vi "CoffeMachineMain.vi"() -> ()   [LabVIEW 2021]
panel:
  in  "Coffe":dbl(slide) scale=0.0..100.0
  in  "Tea":dbl(slide) scale=0.0..100.0
  in  "Water":dbl(slide) scale=0.0..100.0
  in  "İçicek":i64(knob) scale=0.0..2.0
  in  "Sürahi":bool
  in  "Kupa":bool
  out "Preparation":bool
  out "Grinding":bool
  out "Brewing":bool
  out "Distillation":bool
  out "Heating":bool
  out "Cleaning":bool
  out "Status":string
  in  "Power off":bool
  # "Control"
  # "Indıcator"
  # "Tea"
  # "Water"
  # "Coffe"
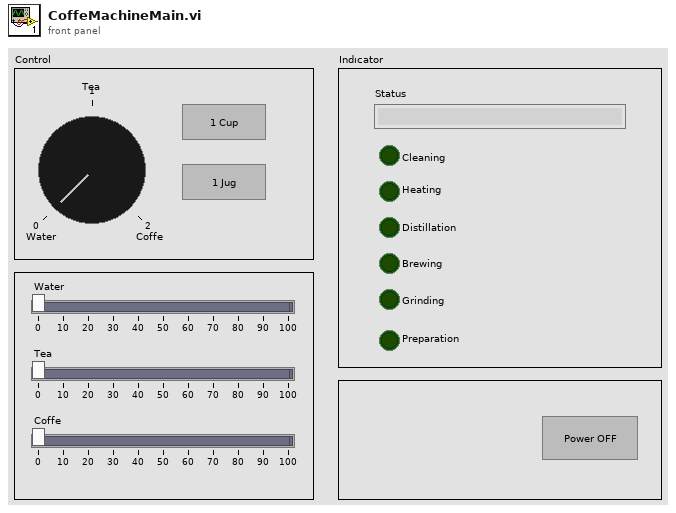
[diagram p1: front panel]
types:
  T1 = cluster{"element":string, "Message Data":variant}
  T2 = cluster{"Çay":dbl, "Su":dbl, "Kahve":dbl, "Power Status":bool}
  T3 = enum8{"Enabled", "Disabled", "Disabled and Grayed Out"}
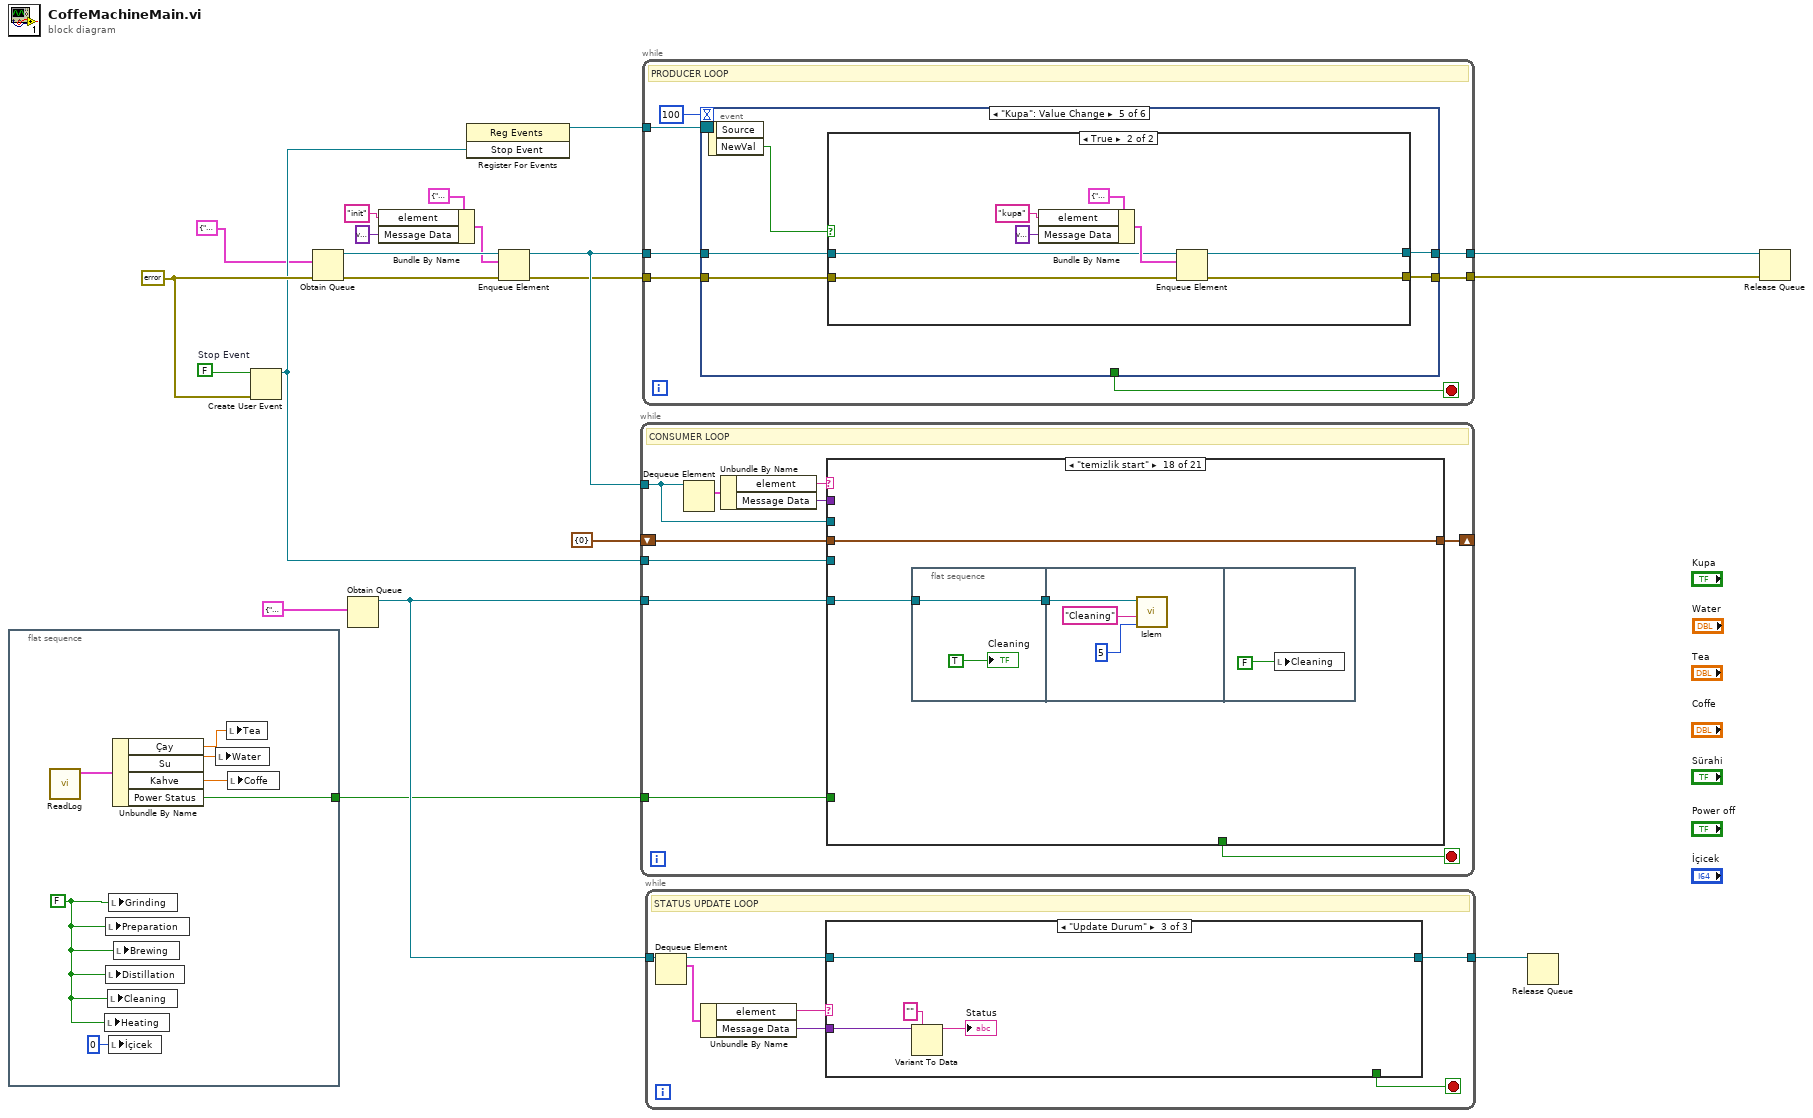
[diagram p0: block diagram]
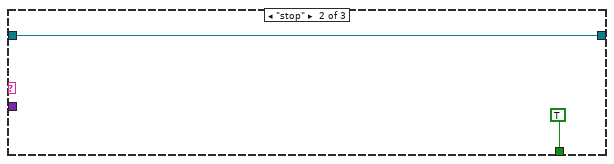
[diagram p3: hidden frame]
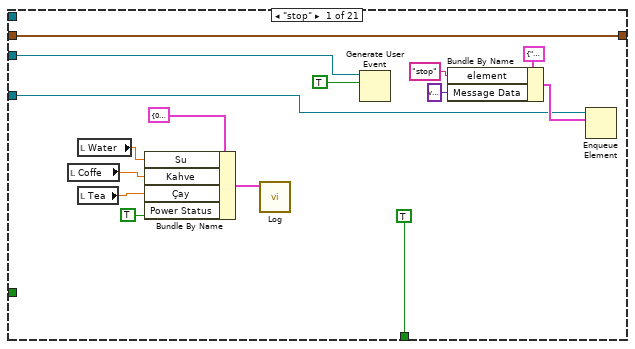
[diagram p4: hidden frame]
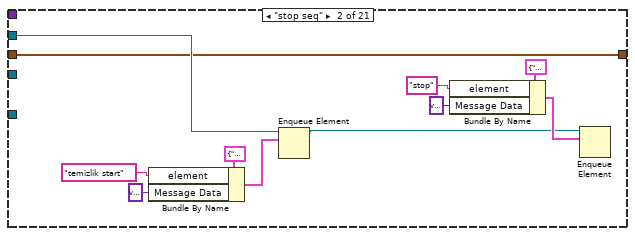
[diagram p5: hidden frame]
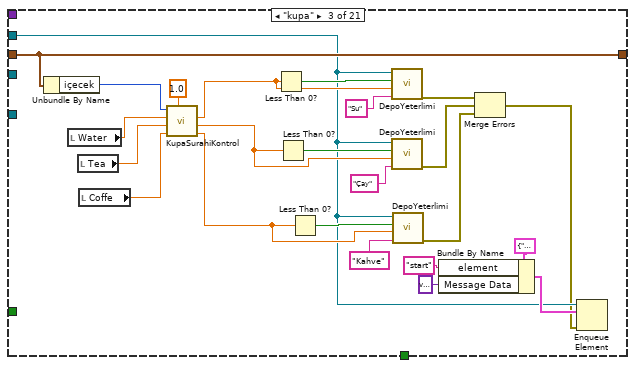
[diagram p6: hidden frame]
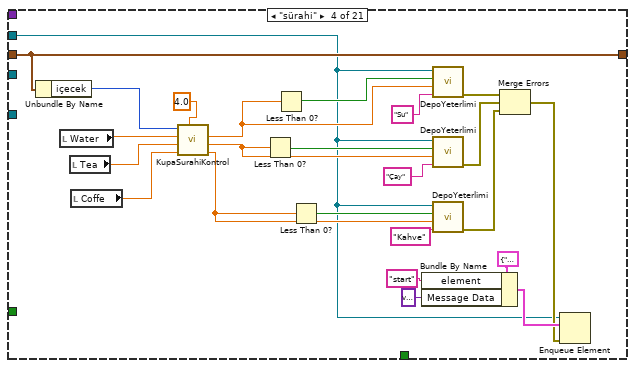
[diagram p7: hidden frame]
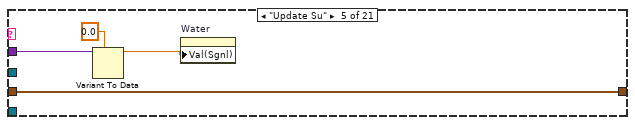
[diagram p8: hidden frame]
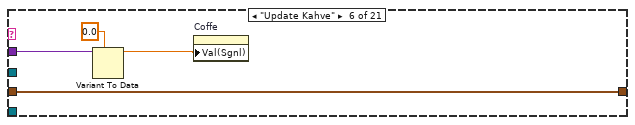
[diagram p9: hidden frame]
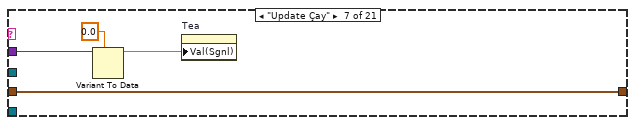
[diagram p10: hidden frame]
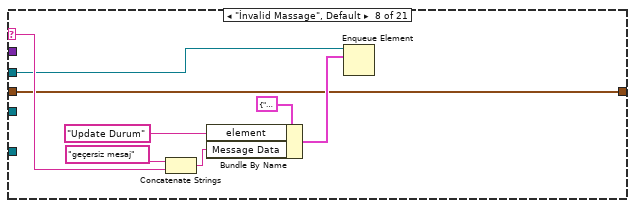
[diagram p11: hidden frame]
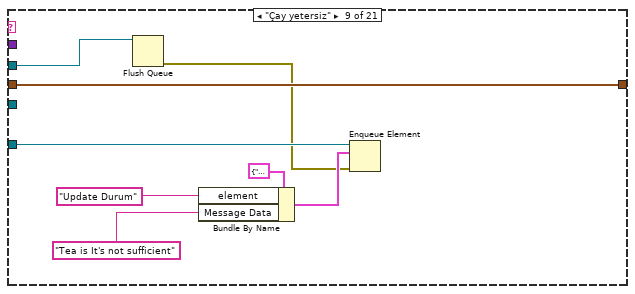
[diagram p12: hidden frame]
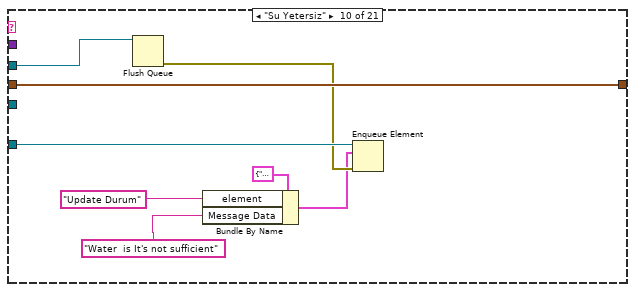
[diagram p13: hidden frame]
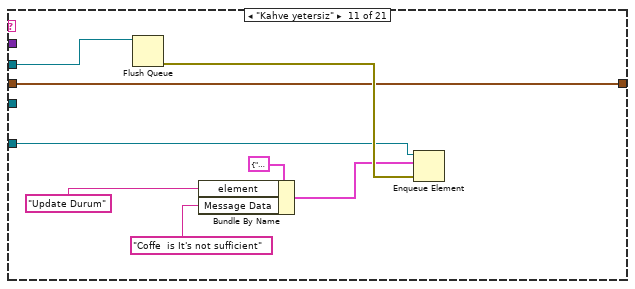
[diagram p14: hidden frame]
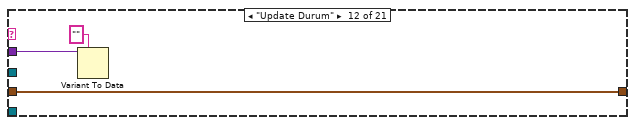
[diagram p15: hidden frame]
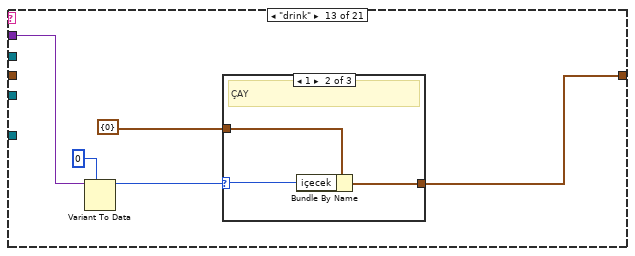
[diagram p16: hidden frame]
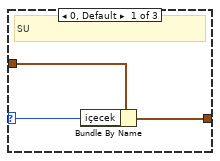
[diagram p17: hidden frame]
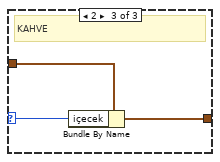
[diagram p18: hidden frame]
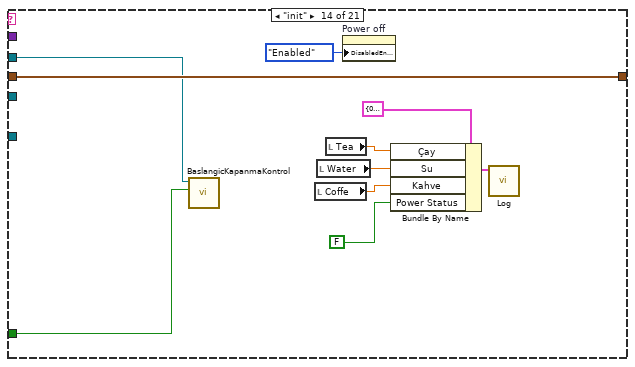
[diagram p19: hidden frame]
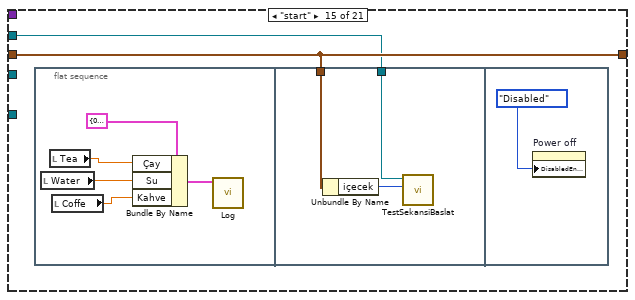
[diagram p20: hidden frame]
diagram:
  w13 = FALSE  # Stop Event
  w14 = errorcluster {"status"=FALSE, "code"=0, "source"=""} ("error in (no error)")
  n1 = flat-sequence {
    tunnel: [w23] -> w1
    frame #0 {
      w22 = FALSE ("Öğütme")
      n2 = call "ReadLog.vi"() -> ("data out"=w27:T2)  [unwired: 11 in]
      n3 = local write "Heating"(w22) -> ()
      n4 = local write "Preparation"(w22) -> ()
      n5 = local write "Distillation"(w22) -> ()
      n6 = local write "Cleaning"(w22) -> ()
      n7 = local write "Grinding"(w22) -> ()
      n8 = local write "İçicek"(i64 0 ("İçicek")) -> ()
      n9 = Unbundle By Name(w27) -> ("Çay"=w25:dbl, "Su"=w26:dbl, "Kahve"=w24:dbl, "Power Status"=w23:bool)
      n10 = local write "Brewing"(w22) -> ()
      n11 = local write "Water"(w26) -> ()
      n12 = local write "Tea"(w25) -> ()
      n13 = local write "Coffe"(w24) -> ()
    }
  }
  n14 = Create User Event(user event datatype=w13, error in=w14) -> (user event=w11:refnum<user-event>)  [unwired: 1 out]
  n15 = Obtain Queue(element data type=T1 {"element"="", "Message Data"=variant}, error in (no error)=w14) -> (queue out=w18:refnum<queue>, error out=w17:errorcluster)  [unwired: 3 in, 1 out]
  n16 = Obtain Queue(element data type=T1 {"element"="", "Message Data"=variant}) -> (queue out=w4:refnum<queue>)  [unwired: 4 in, 2 out]
  n17 = Bundle By Name(cluster=T1 {"element"="", "Message Data"=variant}, "element"="init", "Message Data"=variant) -> (w8:T1)
  n18 = register-events(w11) -> (reference out=w12:refnum<event-registration>)  [unwired: 2 in, 1 out]
  n19 = Enqueue Element(queue=w18, element=w8, error in (no error)=w17) -> (queue out=w16:refnum<queue>, error out=w15:errorcluster)  [unwired: 1 in, 1 out]
  n20 = while {
    tunnel: w16 -> [w30]
    tunnel: w11 -> [w37]
    shift-right: [w32] -> _
    shift-left: cluster{"içecek":i64} {"içecek"=0} -> [w33]
    tunnel: w4 -> [w29]
    tunnel: w1 -> [w28]
    stop <- w36 stop-if-true
    # "CONSUMER LOOP"
    n21 = Dequeue Element(queue=w30) -> (element=w35:T1)  [unwired: 2 in, 3 out]
    n22 = Unbundle By Name(w35) -> ("element"=w34:string, "Message Data"=w31:variant)
    n23 = case shown="\"temizlik start\"" w34 {
      selector: w34 -> [_ _ _ _ _ _ _ w128 _ _ _ _ _ _ _ _ _ _ _ _ _]
      tunnel: w37 -> [w51 _ _ _ _ _ _ _ _ _ _ _ _ _ _ _ _ _ _ _ _]
      tunnel: [TRUE _ _ _ _ _ _ _ _ _ _ _ _ _ _ _ _ _ _ _ _] -> w36
      tunnel: w33 -> [w49 w53 w87 w111 w113 w117 w121 w124 w136 w143 w149 w156 _ w182 w184 w196 w203 w212 w223 w233 w242]
      tunnel: [w49 w53 w87 w111 w113 w117 w121 w124 w136 w143 w149 w156 w160 w182 w184 w196 w203 w212 w223 w233 w242] -> w32
      tunnel: w31 -> [_ _ _ _ w115 w119 w123 _ _ _ _ w158 w163 _ _ _ _ _ _ _ _]
      tunnel: w30 -> [_ w54 w65 w88 _ _ _ w126 w139 w147 w155 _ _ w179 w183 _ _ _ _ _ _]
      tunnel: w29 -> [w44 _ _ _ _ _ _ _ w134 w142 w148 _ _ _ _ w194 w204 w213 w221 w231 w241]
      tunnel: w28 -> [_ _ _ _ _ _ _ _ _ _ _ _ _ w180 _ _ _ _ _ _ _]
      frame "stop" {
        n24 = local read "Coffe"() -> (w40:dbl)
        n25 = local read "Water"() -> (w42:dbl)
        n26 = local read "Tea"() -> (w41:dbl)
        n27 = Bundle By Name(cluster=T2 {"Çay"=0.0, "Su"=0.0, "Kahve"=0.0, "Power Status"=FALSE}, "Su"=w42, "Kahve"=w40, "Çay"=w41, "Power Status"=TRUE) -> (w38:T2)
        n28 = call "Log.vi"("Data"=w38) -> ()  [unwired: 11 in]
        n29 = Generate User Event(user event=w51, event data cluster=TRUE ("event data")) -> ()  [unwired: 2 in, 2 out]
        n30 = Bundle By Name(cluster=T1 {"element"="", "Message Data"=variant}, "element"="stop", "Message Data"=variant) -> (w47:T1)
        n31 = Enqueue Element(queue=w44, element=w47) -> ()  [unwired: 2 in, 3 out]
      }
      frame "stop seq" {
        n32 = Bundle By Name(cluster=T1 {"element"="", "Message Data"=variant}, "element"="temizlik start", "Message Data"=variant) -> (w63:T1)
        n33 = Enqueue Element(queue=w54, element=w63) -> (queue out=w55:refnum<queue>)  [unwired: 2 in, 2 out]
        n34 = Bundle By Name(cluster=T1 {"element"="", "Message Data"=variant}, "element"="stop", "Message Data"=variant) -> (w56:T1)
        n35 = Enqueue Element(queue=w55, element=w56) -> ()  [unwired: 2 in, 3 out]
      }
      frame "kupa" {
        n36 = Unbundle By Name(w87) -> ("içecek"=w85:i64)
        n37 = local read "Water"() -> (w86:dbl)
        n38 = local read "Tea"() -> (w84:dbl)
        n39 = local read "Coffe"() -> (w83:dbl)
        n40 = call "KupaSurahiKontrol.vi"("Çarpan"=1.0, "Kahve"=w83, "Çay"=w84, "Su"=w86, "içicek"=w85) -> ("Kahve çıkış"=w73:dbl, "Çay çıkış"=w76:dbl, "Su çıkış"=w80:dbl)  [unwired: 4 in]
        n41 = Less Than 0?(x=w80) -> (x < 0?=w81:bool)
        n42 = Less Than 0?(x=w76) -> (x < 0?=w77:bool)
        n43 = Less Than 0?(x=w73) -> (x < 0?=w74:bool)
        n44 = call "DepoYeterlimi.vi"("Element"="Su", "Massage Data"=w80, "Yeterlimi?"=w81, "queue out"=w65) -> ("error out"=w72:errorcluster)  [unwired: 7 in]
        n45 = call "DepoYeterlimi.vi"("Element"="Çay", "Massage Data"=w76, "Yeterlimi?"=w77, "queue out"=w65) -> ("error out"=w71:errorcluster)  [unwired: 7 in]
        n46 = call "DepoYeterlimi.vi"("Element"="Kahve", "Massage Data"=w73, "Yeterlimi?"=w74, "queue out"=w65) -> ("error out"=w70:errorcluster)  [unwired: 7 in]
        n47 = Bundle By Name(cluster=T1 {"element"="", "Message Data"=variant}, "element"="start", "Message Data"=variant) -> (w69:T1)
        n48 = Merge Errors(w72, w71, w70) -> (w64:errorcluster)
        n49 = Enqueue Element(queue=w65, element=w69, error in (no error)=w64) -> ()  [unwired: 1 in, 3 out]
      }
      frame "sürahi" {
        n50 = Unbundle By Name(w111) -> ("içecek"=w110:i64)
        n51 = local read "Water"() -> (w108:dbl)
        n52 = local read "Tea"() -> (w107:dbl)
        n53 = local read "Coffe"() -> (w106:dbl)
        n54 = call "KupaSurahiKontrol.vi"("Çarpan"=4.0 ("x"), "Kahve"=w106, "Çay"=w107, "Su"=w108, "içicek"=w110) -> ("Kahve çıkış"=w97:dbl, "Çay çıkış"=w100:dbl, "Su çıkış"=w104:dbl)  [unwired: 4 in]
        n55 = Less Than 0?(x=w100) -> (x < 0?=w101:bool)
        n56 = Less Than 0?(x=w104) -> (x < 0?=w105:bool)
        n57 = Less Than 0?(x=w97) -> (x < 0?=w98:bool)
        n58 = Bundle By Name(cluster=T1 {"element"="", "Message Data"=variant}, "element"="start", "Message Data"=variant) -> (w93:T1)
        n59 = call "DepoYeterlimi.vi"("Element"="Su" ("element"), "Massage Data"=w104, "Yeterlimi?"=w105, "queue out"=w88) -> ("error out"=w96:errorcluster)  [unwired: 7 in]
        n60 = call "DepoYeterlimi.vi"("Element"="Çay" ("element"), "Massage Data"=w100, "Yeterlimi?"=w101, "queue out"=w88) -> ("error out"=w95:errorcluster)  [unwired: 7 in]
        n61 = call "DepoYeterlimi.vi"("Element"="Kahve", "Massage Data"=w97, "Yeterlimi?"=w98, "queue out"=w88) -> ("error out"=w94:errorcluster)  [unwired: 7 in]
        n62 = Merge Errors(w96, w95, w94) -> (w89:errorcluster)
        n63 = Enqueue Element(queue=w88, element=w93, error in (no error)=w89) -> ()  [unwired: 1 in, 3 out]
      }
      frame "Update Su" {
        n64 = Variant To Data(type=0.0 ("Su"), Variant=w115) -> (data=w112:dbl)  [unwired: 1 in, 1 out]
        n65 = property on="Water" class="Slide (strict)"("Val(Sgnl)"=w112) -> ()  [unwired: 2 in, 2 out]
      }
      frame "Update Kahve" {
        n66 = Variant To Data(type=0.0 ("Su"), Variant=w119) -> (data=w116:dbl)  [unwired: 1 in, 1 out]
        n67 = property on="Coffe" class="Slide (strict)"("Val(Sgnl)"=w116) -> ()  [unwired: 2 in, 2 out]
      }
      frame "Update Çay" {
        n68 = Variant To Data(type=0.0 ("Su"), Variant=w123) -> (data=w120:dbl)  [unwired: 1 in, 1 out]
        n69 = property on="Tea" class="Slide (strict)"("Val(Sgnl)"=w120) -> ()  [unwired: 2 in, 2 out]
      }
      frame "İnvalid Massage", Default {
        n70 = Concatenate Strings("geçersiz mesaj" ("element"), w128) -> (w127:string)
        n71 = Bundle By Name(cluster=T1 {"element"="", "Message Data"=variant}, "element"="Update Durum", "Message Data"=w127) -> (w125:T1)
        n72 = Enqueue Element(queue=w126, element=w125) -> ()  [unwired: 2 in, 3 out]
      }
      frame "Çay yetersiz" {
        n73 = Flush Queue(queue=w139) -> (error out=w132:errorcluster)  [unwired: 1 in, 2 out]
        n74 = Bundle By Name(cluster=T1 {"element"="", "Message Data"=variant}, "element"="Update Durum", "Message Data"="Tea is It's not sufficient" ("element")) -> (w133:T1)
        n75 = Enqueue Element(queue=w134, element=w133, error in (no error)=w132) -> ()  [unwired: 1 in, 3 out]
      }
      frame "Su Yetersiz" {
        n76 = Flush Queue(queue=w147) -> (error out=w141:errorcluster)  [unwired: 1 in, 2 out]
        n77 = Bundle By Name(cluster=T1 {"element"="", "Message Data"=variant}, "element"="Update Durum", "Message Data"="Water  is It's not sufficient" ("element")) -> (w140:T1)
        n78 = Enqueue Element(queue=w142, element=w140, error in (no error)=w141) -> ()  [unwired: 1 in, 3 out]
      }
      frame "Kahve yetersiz" {
        n79 = Flush Queue(queue=w155) -> (error out=w154:errorcluster)  [unwired: 1 in, 2 out]
        n80 = Bundle By Name(cluster=T1 {"element"="", "Message Data"=variant}, "element"="Update Durum", "Message Data"="Coffe  is It's not sufficient" ("element")) -> (w151:T1)
        n81 = Enqueue Element(queue=w148, element=w151, error in (no error)=w154) -> ()  [unwired: 1 in, 3 out]
      }
      frame "Update Durum" {
        n82 = Variant To Data(type="" ("element"), Variant=w158) -> ()  [unwired: 1 in, 2 out]
      }
      frame "drink" {
        n83 = Variant To Data(type=i64 0 ("NewVal"), Variant=w163) -> (data=w161:i64)  [unwired: 1 in, 1 out]
        n84 = case shown="1" w161 {
          selector: w161 -> [w164 w167 w170]
          tunnel: [w165 w168 w171] -> w160
          tunnel: cluster{"içecek":i64} {"içecek"=0} -> [w166 w169 w172]
          frame 0, Default {
            # "SU"
            n85 = Bundle By Name(cluster=w166, "içecek"=w164) -> (w165:cluster{"içecek":i64})
          }
          frame 1 {
            # "ÇAY"
            n86 = Bundle By Name(cluster=w169, "içecek"=w167) -> (w168:cluster{"içecek":i64})
          }
          frame 2 {
            # "KAHVE"
            n87 = Bundle By Name(cluster=w172, "içecek"=w170) -> (w171:cluster{"içecek":i64})
          }
        }
      }
      frame "init" {
        n88 = call "BaslangicKapanmaKontrol.vi"("Normal Kapanma"=w180, "queue"=w179) -> ()  [unwired: 10 in]
        n89 = local read "Coffe"() -> (w175:dbl)
        n90 = local read "Water"() -> (w176:dbl)
        n91 = local read "Tea"() -> (w177:dbl)
        n92 = property on="Power off" class="Bool"("DisabledEnum"=T3."Enabled" ("Disabled")) -> ()  [unwired: 2 in, 2 out]
        n93 = Bundle By Name(cluster=T2 {"Çay"=0.0, "Su"=0.0, "Kahve"=0.0, "Power Status"=FALSE}, "Çay"=w177, "Su"=w176, "Kahve"=w175, "Power Status"=FALSE) -> (w178:T2)
        n94 = call "Log.vi"("Data"=w178) -> ()  [unwired: 11 in]
      }
      frame "start" {
        n95 = flat-sequence {
          tunnel: w184 -> [w192]
          tunnel: w183 -> [w190]
          frame #0 {
            n96 = local read "Water"() -> (w186:dbl)
            n97 = local read "Tea"() -> (w187:dbl)
            n98 = local read "Coffe"() -> (w185:dbl)
            n99 = Bundle By Name(cluster=T2 {"Çay"=0.0, "Su"=0.0, "Kahve"=0.0, "Power Status"=FALSE}, "Çay"=w187, "Su"=w186, "Kahve"=w185) -> (w188:T2)
            n100 = call "Log.vi"("Data"=w188) -> ()  [unwired: 11 in]
          }
          frame #1 {
            n101 = Unbundle By Name(w192) -> ("içecek"=w191:i64)
            n102 = call "TestSekansiBaslat.vi"("içecek"=w191, "queue in"=w190) -> ()  [unwired: 10 in]
          }
          frame #2 {
            n103 = property on="Power off" class="Bool"("DisabledEnum"=T3."Disabled" ("Disabled")) -> ()  [unwired: 2 in, 2 out]
          }
        }
      }
      frame "ogutme start" {
        n104 = flat-sequence {
          tunnel: [w198] -> w195
          tunnel: w194 -> [w198]
          tunnel: w195 -> [w201]
          frame #0 {
            "Grinding" <- TRUE ("Damitma")
          }
          frame #1 {
            n105 = call "Islem.vi"("Wait time(s)"=5, "İşlem"="Grinding", "queue"=w201) -> ()  [unwired: 9 in]
          }
          frame #2 {
            n106 = local write "Grinding"(FALSE ("Damitma")) -> ()
          }
        }
      }
      frame "isitma start" {
        n107 = flat-sequence {
          tunnel: [w207] -> w205
          tunnel: w204 -> [w207]
          tunnel: w205 -> [w210]
          frame #0 {
            "Heating" <- TRUE ("Damitma")
          }
          frame #1 {
            n108 = call "Islem.vi"("Wait time(s)"=7, "İşlem"="Heating", "queue"=w210) -> ()  [unwired: 9 in]
          }
          frame #2 {
            n109 = local write "Heating"(FALSE ("Damitma")) -> ()
          }
        }
      }
      frame "temizlik start" {
        n110 = flat-sequence {
          tunnel: [w216] -> w214
          tunnel: w213 -> [w216]
          tunnel: w214 -> [w219]
          frame #0 {
            "Cleaning" <- TRUE ("Damitma")
          }
          frame #1 {
            n111 = call "Islem.vi"("Wait time(s)"=5, "İşlem"="Cleaning", "queue"=w219) -> ()  [unwired: 9 in]
          }
          frame #2 {
            n112 = local write "Cleaning"(FALSE ("Damitma")) -> ()
          }
        }
      }
      frame "hazirlama start" {
        n113 = flat-sequence {
          tunnel: [w225] -> w222
          tunnel: w221 -> [w225]
          tunnel: w222 -> [w228]
          frame #0 {
            "Preparation" <- TRUE ("Damitma")
          }
          frame #1 {
            n114 = call "Islem.vi"("Wait time(s)"=3, "İşlem"="Preparation", "queue"=w228) -> ()  [unwired: 9 in]
          }
          frame #2 {
            n115 = local write "Preparation"(FALSE ("Damitma")) -> ()
          }
          frame #3 {
            n116 = property on="Power off" class="Bool"("DisabledEnum"=T3."Enabled" ("Disabled")) -> ()  [unwired: 2 in, 2 out]
          }
        }
      }
      frame "damitma start" {
        n117 = flat-sequence {
          tunnel: [w235] -> w232
          tunnel: w231 -> [w235]
          tunnel: w232 -> [w238]
          frame #0 {
            "Distillation" <- TRUE ("Damitma")
          }
          frame #1 {
            n118 = call "Islem.vi"("Wait time(s)"=3, "İşlem"="Distillation", "queue"=w238) -> ()  [unwired: 9 in]
          }
          frame #2 {
            n119 = local write "Distillation"(FALSE ("Damitma")) -> ()
          }
        }
      }
      frame "demleme start" {
        n120 = flat-sequence {
          tunnel: w241 -> [w243]
          tunnel: [w243] -> w240
          tunnel: w240 -> [w245]
          frame #0 {
            "Brewing" <- TRUE ("Damitma")
          }
          frame #1 {
            n121 = call "Islem.vi"("Wait time(s)"=7, "İşlem"="Brewing", "queue"=w245) -> ()  [unwired: 9 in]
          }
          frame #2 {
            n122 = local write "Brewing"(FALSE ("Damitma")) -> ()
          }
        }
      }
    }
  }
  n123 = while {
    tunnel: w16 -> [w255]
    tunnel: [w253] -> w20
    tunnel: w15 -> [w254]
    tunnel: [w252] -> w19
    tunnel: w12 -> [w251]
    stop <- w250 stop-if-true
    # "PRODUCER LOOP"
    n124 = event shown="[4] \"Kupa\": Value Change" {
      selector: w251 -> [_ _ _ _ _ _]
      dyn-events: _ -> [_ _ _ _ _ _]
      timeout: 100 -> [_ _ _ _ _ _]
      tunnel: w255 -> [w261 w269 w271 w280 w285 w300]
      tunnel: w254 -> [w260 w268 w270 w278 w284 w299]
      tunnel: [w261 w266 w271 w279 w283 w298] -> w253
      tunnel: [w260 w267 w270 w277 w282 w297] -> w252
      tunnel: [_ _ TRUE _ _ _] -> w250
      event Timeout {
        n125 = event-data() -> ()  [unwired: 1 in, 3 out]
        n126 = local read "Water"() -> (w259:dbl)
        n127 = local read "Tea"() -> (w258:dbl)
        n128 = local read "Coffe"() -> (w257:dbl)
        n129 = call "Yuzde30Kontrol.vi"("Kahve"=w257, "Çay"=w258, "Su"=w259) -> ("Disabled"=w256:T3)  [unwired: 8 in]
        n130 = property on="Kupa" class="Bool"("DisabledEnum"=w256) -> ()  [unwired: 2 in, 2 out]
        n131 = property on="Sürahi" class="Bool (strict)"("DisabledEnum"=w256) -> ()  [unwired: 2 in, 2 out]
      }
      event "Power off": Value Change {
        n132 = event-data() -> ()  [unwired: 1 in, 1 out]
        n133 = Bundle By Name(cluster=T1 {"element"="", "Message Data"=variant}, "element"="stop seq", "Message Data"=variant) -> (w262:T1)
        n134 = Enqueue Element(queue=w269, element=w262, error in (no error)=w268) -> (queue out=w266:refnum<queue>, error out=w267:errorcluster)  [unwired: 1 in, 1 out]
      }
      event User Event {
        n135 = event-data() -> ()  [unwired: 1 in, 5 out]
      }
      event "İçicek": Value Change {
        n136 = event-data() -> ("NewVal"=w273:i64)  [unwired: 1 in, 5 out]
        n137 = Bundle By Name(cluster=T1 {"element"="", "Message Data"=variant}, "element"="drink", "Message Data"=w273) -> (w274:T1)
        n138 = Enqueue Element(queue=w280, element=w274, error in (no error)=w278) -> (queue out=w279:refnum<queue>, error out=w277:errorcluster)  [unwired: 1 in, 1 out]
      }
      event "Kupa": Value Change {
        n139 = event-data() -> ("NewVal"=w281:bool)  [unwired: 1 in, 1 out]
        n140 = case shown="True" w281 {
          tunnel: w285 -> [w286 w291]
          tunnel: w284 -> [w287 w290]
          tunnel: [w286 w289] -> w283
          tunnel: [w287 w288] -> w282
          frame False {
          }
          frame True {
            n141 = Bundle By Name(cluster=T1 {"element"="", "Message Data"=variant}, "element"="kupa", "Message Data"=variant) -> (w293:T1)
            n142 = Enqueue Element(queue=w291, element=w293, error in (no error)=w290) -> (queue out=w289:refnum<queue>, error out=w288:errorcluster)  [unwired: 1 in, 1 out]
          }
        }
      }
      event "Sürahi": Value Change {
        n143 = event-data() -> ("NewVal"=w296:bool)  [unwired: 1 in, 1 out]
        n144 = case shown="True" w296 {
          tunnel: w300 -> [w302 w306]
          tunnel: w299 -> [w301 w305]
          tunnel: [w302 w304] -> w298
          tunnel: [w301 w303] -> w297
          frame False {
          }
          frame True {
            n145 = Bundle By Name(cluster=T1 {"element"="", "Message Data"=variant}, "element"="sürahi", "Message Data"=variant) -> (w308:T1)
            n146 = Enqueue Element(queue=w306, element=w308, error in (no error)=w305) -> (queue out=w304:refnum<queue>, error out=w303:errorcluster)  [unwired: 1 in, 1 out]
          }
        }
      }
    }
  }
  n147 = while {
    tunnel: w4 -> [w315]
    tunnel: [w311] -> w3
    stop <- w313 stop-if-true
    # "STATUS UPDATE LOOP"
    n148 = Dequeue Element(queue=w315) -> (queue out=w312:refnum<queue>, element=w314:T1)  [unwired: 2 in, 2 out]
    n149 = Unbundle By Name(w314) -> ("element"=w317:string, "Message Data"=w316:variant)
    n150 = case shown="\"Update Durum\"" w317 {
      tunnel: w316 -> [_ _ w322]
      tunnel: [_ TRUE _] -> w313
      tunnel: w312 -> [w318 w319 w321]
      tunnel: [w318 w319 w321] -> w311
      frame "False", Default {
      }
      frame "stop" {
      }
      frame "Update Durum" {
        n151 = Variant To Data(type="" ("element"), Variant=w322) -> (data=→"Status":string)  [unwired: 1 in, 1 out]
      }
    }
  }
  n152 = Release Queue(queue=w3) -> ()  [unwired: 2 in, 3 out]
  n153 = Release Queue(queue=w20, error in (no error)=w19) -> ()  [unwired: 1 in, 3 out]
